vi "idn.vi"(6 "timeout (ms)":i32=10000, 7 "IP address":string, 8 "error in (no error)":errorcluster, 9 "token cluster in":T1, 11 "client handle":T2) -> (0 "error out":errorcluster, 1 "token cluster":T1, 2 "idn":string, 3 "client handle out":T2)   [LabVIEW 2018]
uses:
  <vilib>/httpClient/ClientHandle.ctl
  <vilib>/httpClient/LabVIEWHTTPClient.lvlib
panel:
  out "headers":string
  out "status code":string
  out "msg":string
  out "reponse":string
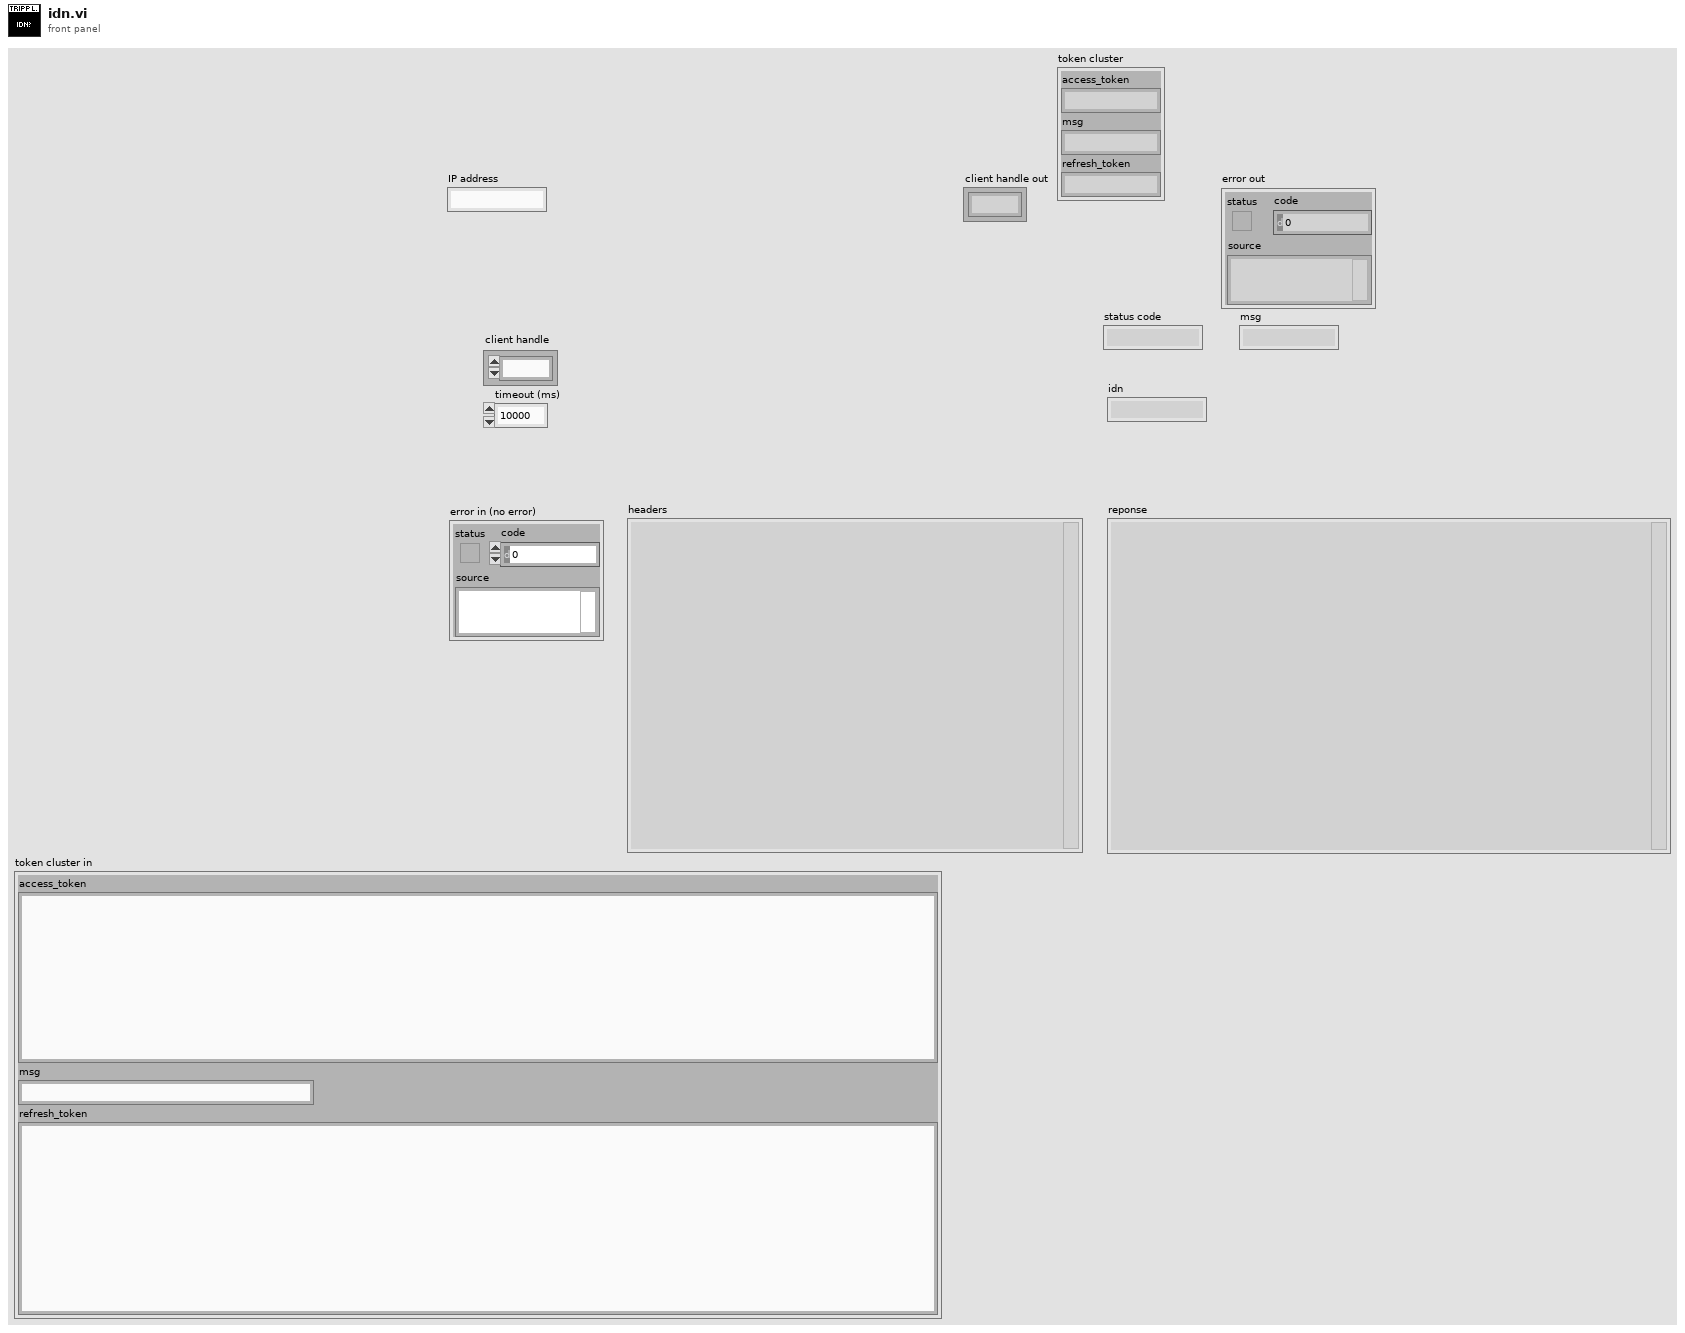
[diagram p1: front panel]
types:
  T1 = cluster{"access_token":string, "msg":string, "refresh_token":string}
  T2 = typedef "LabVIEWHTTPClient.lvlib/ClientHandle.ctl" = refnum<k1>
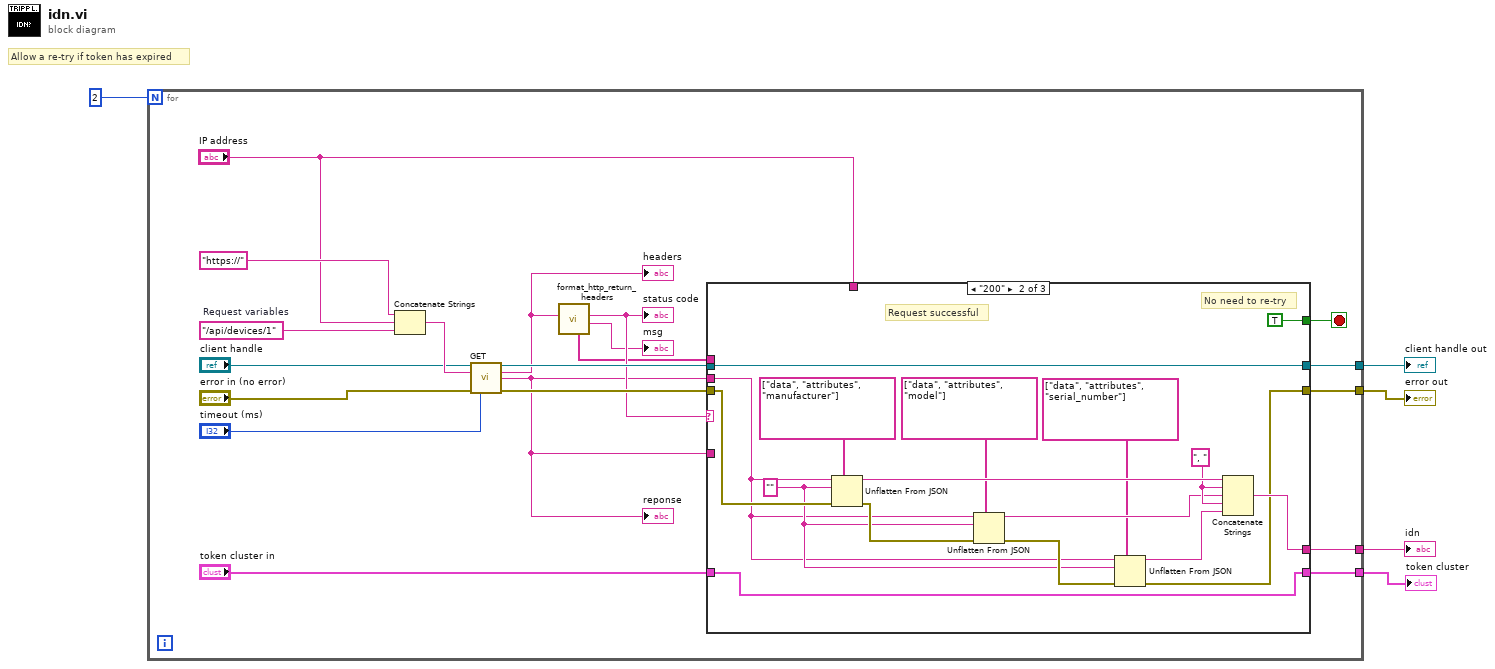
[diagram p0: block diagram]
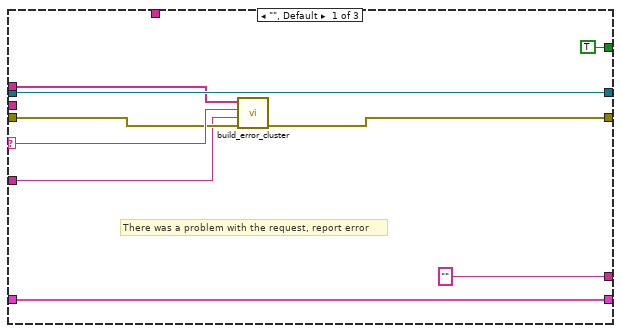
[diagram p2: hidden frame]
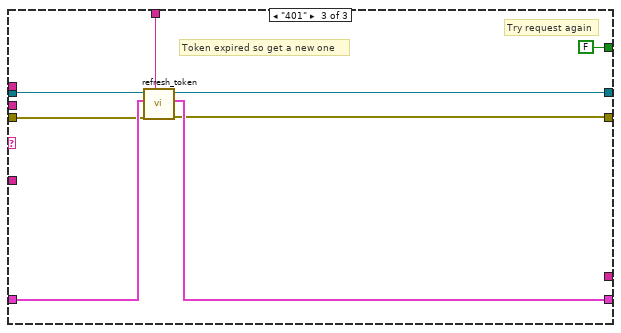
[diagram p3: hidden frame]
diagram:
  # "Allow a re-try if token has expired"
  n1 = for {
    N: 2 -> [_]
    tunnel: [w20] -> w5
    tunnel: [w19] -> w4
    tunnel: [w11] -> w3
    tunnel: [w8] -> w2
    stop <- w6 stop-if-true
    w22 = "/api/devices/1"  # Request variables
    n2 = Concatenate Strings("https://", "IP address", w22) -> (w25:string)
    n3 = call <vilib>:"GET.vi"("client handle"="client handle", "url"=w25, "error in (no error)"="error in (no error)", "timeout (10000)"="timeout (ms)") -> ("client handle out"=w23:T2, "headers"=w18:string, "body"=w10:string, "error out"=w24:errorcluster)  [unwired: 8 in]
    "reponse" <- w10
    "headers" <- w18
    n4 = call "format_http_return_headers.vi"("headers in"=w18) -> ("msg"=→"msg":string, "status code"=w17:string, "headers array"=w15:string[])  [unwired: 8 in]
    "status code" <- w17
    n5 = case shown="\"200\"" w17 {
      selector: w17 -> [w33 _ _]
      tunnel: w24 -> [w31 w50 w55]
      tunnel: w10 -> [_ w46 _]
      tunnel: w23 -> [w34 w51 w57]
      tunnel: [w30 w39 w54] -> w20
      tunnel: [w34 w51 w56] -> w19
      tunnel: ["" ("body") w40 _] -> w11
      tunnel: w15 -> [w32 _ _]
      tunnel: w10 -> [w28 _ _]
      tunnel: "token cluster in" -> [w27 w36 w59]
      tunnel: [w27 w36 w58] -> w8
      tunnel: "IP address" -> [_ _ w53]
      tunnel: [TRUE TRUE FALSE] -> w6
      frame "", Default {
        # "There was a problem with the request, report error"
        n6 = call "build_error_cluster.vi"("error in (no error)"=w31, "error msg (JSON)"=w28, "status code"=w33, "headers array"=w32) -> ("error out"=w30:errorcluster)  [unwired: 7 in]
      }
      frame "200" {
        w43 = ", "
        w47 = ""
        # "No need to re-try"
        # "Request successful"
        n7 = Unflatten From JSON(path=string[] ["data", "attributes", "manufacturer"], JSON string=w46, type and defaults=w47, error in (no error)=w50) -> (value=w44:string, error out=w49:errorcluster)  [unwired: 3 in]
        n8 = Unflatten From JSON(path=string[] ["data", "attributes", "model"], JSON string=w46, type and defaults=w47, error in (no error)=w49) -> (value=w42:string, error out=w48:errorcluster)  [unwired: 3 in]
        n9 = Unflatten From JSON(path=string[] ["data", "attributes", "serial_number"], JSON string=w46, type and defaults=w47, error in (no error)=w48) -> (value=w41:string, error out=w39:errorcluster)  [unwired: 3 in]
        n10 = Concatenate Strings(w44, w43, w42, w43, w41) -> (w40:string)
      }
      frame "401" {
        # "Try request again"
        # "Token expired so get a new one"
        n11 = call "refresh_token.vi"("IP address"=w53, "error in (no error)"=w55, "token cluster in"=w59, "client handle"=w57) -> ("error out"=w54:errorcluster, "token cluster"=w58:T1, "client handle out"=w56:T2)  [unwired: 5 in]
      }
    }
  }
  "error out" <- w5
  "client handle out" <- w4
  "idn" <- w3
  "token cluster" <- w2
